vi "Disable_and_Start.vi"(8 "error in (no error)":errorcluster, 9 "Underbody Wash":refnum<vi>, 10 "Data":variant, 11 "System data in":T1) -> (0 "error out":errorcluster, 3 "System data out":T1)   [LabVIEW 2023]
doc: "This VI ddiables the car wash options and starts the washing process"
uses:
  Controls/System_Data.ctl
  Controls/Wash Options.ctl
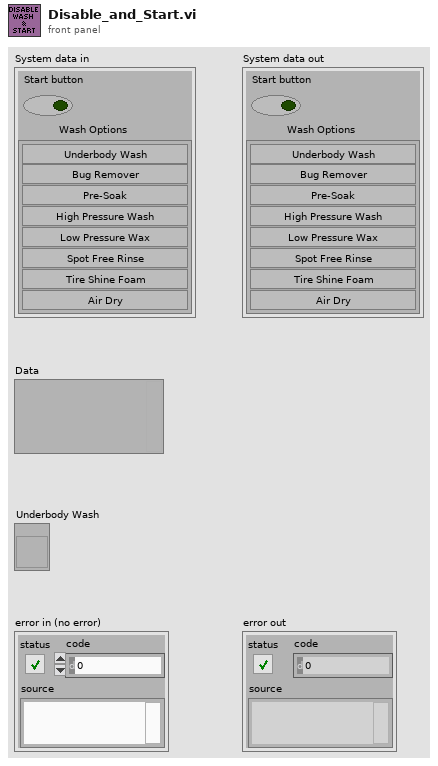
[diagram p1: front panel]
types:
  T1 = typedef "System_Data.ctl" = cluster{"Start button":bool, "Wash Options":T2}
  T2 = typedef "Wash Options.ctl" = cluster{"Underbody Wash":bool, "Bug Remover":bool, "Pre-Soak":bool, "High Pressure Wash":bool, "Low Pressure Wax":bool, "Spot Free Rinse":bool, "Tire Shine Foam":bool, "Air Dry":bool}
  T3 = enum8{"Enabled", "Disabled", "Disabled and Grayed Out"}
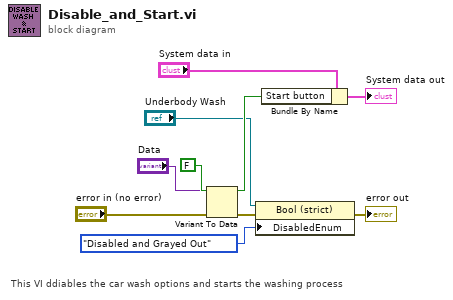
[diagram p0: block diagram]
diagram:
  # "This VI ddiables the car wash options and starts the washing process"
  n1 = Variant To Data(error in="error in (no error)", type=FALSE, Variant="Data") -> (data=w9:bool, error out=w10:errorcluster)
  n2 = property class="Bool (strict)"(reference="Underbody Wash", error in=w10, "DisabledEnum"=T3."Disabled and Grayed Out" ("Disabled")) -> (error out=→"error out":errorcluster)  [unwired: 1 out]
  n3 = Bundle By Name(cluster="System data in", "Start button"=w9) -> (→"System data out":T1)
